vi "get_aw_tune.vi"(6 "timeout (25000ms)":i32=25000, 8 "error in (no error)":errorcluster, 10 "Index":u32 max=5, 11 "daemon reference in":refnum<k5>) -> (0 "error out":errorcluster, 1 "AW Tune Parameter":T1, 2 "response":string, 3 "daemon reference out":refnum<k5>, 5 "command out":string="random")   [LabVIEW 2017]
doc: "<b>Command: </b>\"get_aw_tune\"\n\n<b>Description: </b> Gets the airwatts delta power tuning parameter for the desired power mode.\n\n<b>Parameters: </b> Index (0-5)\n____________________________________________\nDIPC 692 Daemon API 10.0.0.1\nSam Tee - Dyson Technology Ltd\nCopyright (c) 2024, Dyson Technology Ltd"
uses:
  typdef/airwatt tune parameter.ctl
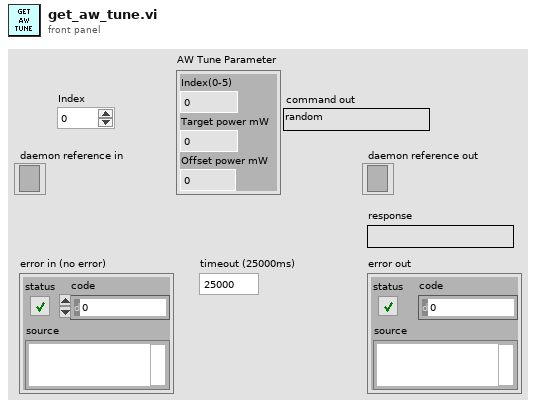
[diagram p1: front panel]
types:
  T1 = typedef "airwatt tune parameter.ctl" = cluster{"Index(0-5)":i64, "Target power mW":i64, "Offset power mW":i64}
  T2 = cluster{"array type (2D Dbl)[0]":dbl, "array type (2D Dbl)[1]":dbl, "array type (2D Dbl)[2]":dbl}
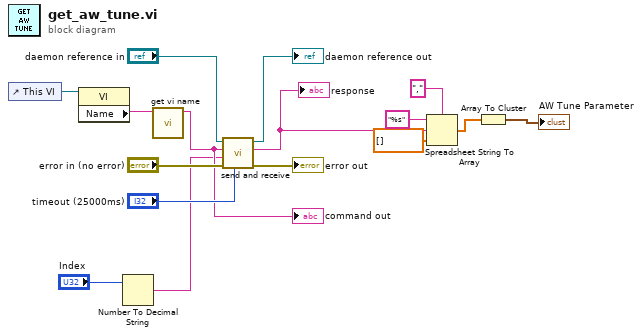
[diagram p0: block diagram]
diagram:
  n1 = control-ref of="This VI"() -> (w11:refnum<vi>)
  n2 = property class="VI"(reference=w11) -> ("Name"=w10:string)  [unwired: 1 in, 2 out]
  n3 = Number To Decimal String(number="Index") -> (decimal integer string=w7:string)  [unwired: 1 in]
  n4 = call "get vi name.vi"("library.lvlib:name.vi"=w10) -> ("vi name"=w9:string)  [unwired: 10 in]
  "command out" <- w9
  n5 = call "send and receive.vi"("timeout (25000ms)"="timeout (25000ms)", "error in (no error)"="error in (no error)", "data"=w7, "command"=w9, "daemon reference in"="daemon reference in") -> ("error out"=→"error out":errorcluster, "response"=w5:string, "daemon reference out"=→"daemon reference out":refnum<k5>)  [unwired: 4 in]
  "response" <- w5
  n6 = Spreadsheet String To Array(delimiter (Tab)=",", format string="%s", spreadsheet string=w5, array type (2D Dbl)=dbl[] []) -> (array=w2:dbl[])
  n7 = Array To Cluster(array=w2) -> (cluster=→"AW Tune Parameter":T2)
